vi "hexatodecimal1 (SubVI).vi"(11 "string in":string) -> (3 "Numeric":u32)   [LabVIEW 2015]
panel:
  out "after substring":string
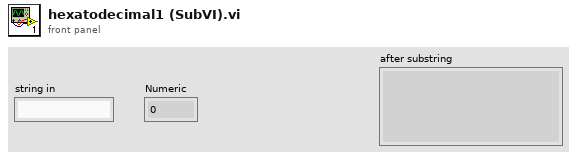
[diagram p1: front panel]
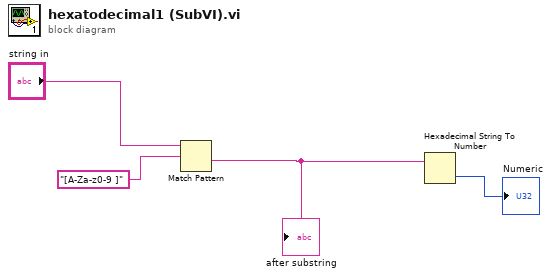
[diagram p0: block diagram]
diagram:
  n1 = Match Pattern(string="string in", regular expression="[A-Za-z0-9 ]") -> (after substring=w2:string)  [unwired: 1 in, 3 out]
  "after substring" <- w2
  n2 = Hexadecimal String To Number(string=w2) -> (number=→"Numeric":u32)  [unwired: 2 in, 1 out]
